vi "ExSetupROI.vi"() -> ()   [LabVIEW 2010]
uses:
  Open-Close Hardware/CamHandle.vi
panel:
  out "frames":u32=5341
  out "ADC Speed":u32=20000
  out "error out":errorcluster
  in  "error in (no error)":errorcluster
  in  "Timing Mode":u32(ring)=1 items=["N/A", "Timed Mode/Free run", "Trigger First (only PM)", "Strobed/Ext Sync", "Bulb Mode (PM only)", "Variable Timed mode (PM only)", "Flash Mode (only some PM)"]
  in  "x1":u32=1
  in  "x2":u32=256
  in  "y1":u32=1
  in  "y2":u32=256
  in  "x bin":u32=1
  in  "y bin":u32=1
  in  "min block":u32=2
  in  "Num Min Block":u32=5
  # "ExSetupROI.vi : This vi setups up 1 ROI (Region Of Interest)."
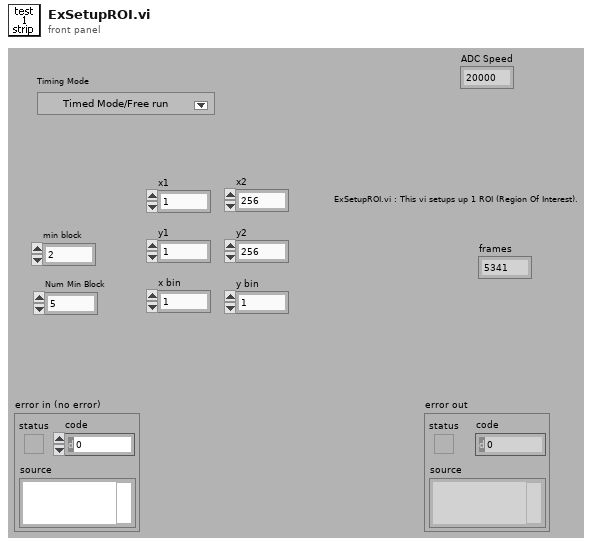
[diagram p1: front panel]
types:
  T1 = cluster{"x1":u32, "x2":u32, "x bin":u32, "y1":u32, "y2":u32, "y bin":u32}
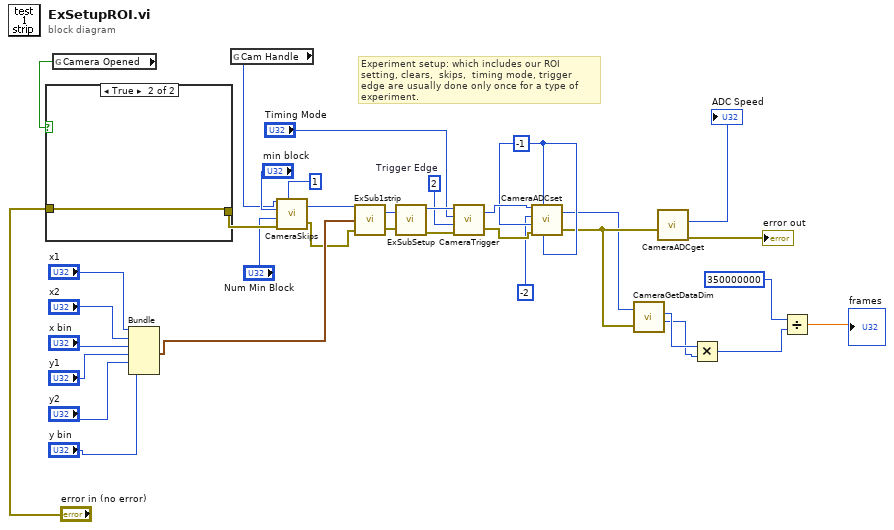
[diagram p0: block diagram]
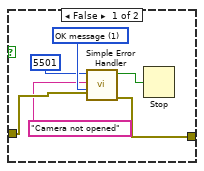
[diagram p2: hidden frame]
diagram:
  w29 = -1
  w33 = u32 2  # Trigger Edge
  # "Experiment setup: which includes our ROI setting, clears,  skips,  timing mode, trigger edge are usually done only once for a type of experiment."
  n1 = global read "CamHandle.vi" "Camera Opened"() -> (w32:bool)
  n2 = case shown="True" w32 {
    tunnel: "error in (no error)" -> [w40 w42]
    tunnel: [w39 w42] -> w19
    frame False {
      w41 = u16 1 items=["no dialog", "OK message", "continue or stop message"] ("type of dialog (OK msg:1)")
      n3 = call <vilib>:"Simple Error Handler.vi"("error code (no error:0)"=5501, "error source (\" \")"="Camera not opened", "type of dialog (OK msg:1)"=w41, "error in (no error)"=w40) -> ("error?"=w37:bool, "error out"=w39:errorcluster)  [unwired: 1 in, 3 out]
      n4 = Stop(stop? (T)=w37) -> ()
    }
    frame True {
    }
  }
  n5 = Bundle("x1"="x1", "x2"="x2", "x bin"="x bin", "y1"="y1", "y2"="y2", "y bin"="y bin") -> (w20:T1)  [unwired: 1 in]
  n6 = global read "CamHandle.vi" "Cam Handle"() -> (w12:u32)
  n7 = call <userlib>:"CameraSkips.vi"("Camera Handle"=w12, "Minimum Block Size"="min block", "Number of Minimum blocks"="Num Min Block", "error in"=w19, "Type of Skips"=1) -> ("Camera Handle"=w17:u32, "error out"=w18:errorcluster)
  n8 = call "ExSub1strip.vi"("error in (no error)"=w18, "strip 1"=w20, "Camera Handle"=w17) -> ("error out"=w27:errorcluster, "Camera Handle"=w13:u32)
  n9 = call "ExSubSetup.vi"("error in (no error)"=w27, "Camera Handle"=w13) -> ("error out"=w34:errorcluster, "Camera Handle"=w35:u32)
  n10 = call <userlib>:"CameraTrigger.vi"("error in"=w34, "Trigger Edge"=w33, "Timing Mode"="Timing Mode", "Camera Handle"=w35) -> ("error out"=w31:errorcluster, "Camera Handle"=w30:u32)
  n11 = call <userlib>:"CameraADCset.vi"("ADC offset"=w29, "Read Out port"=w29, "error in (no error)"=w31, "ADC Gain"=w29, "ADC Speed"=-2, "Camera Handle"=w30) -> ("error out"=w7:errorcluster, "Camera Handle"=w6:u32)
  n12 = call <userlib>:"CameraGetDataDim.vi"("Camera Handle"=w6, "error in"=w7) -> ("Xdim"=w5:u32, "Ydim"=w4:u32)  [unwired: 2 out]
  n13 = call <userlib>:"CameraADCget.vi"("error in (no error)"=w7) -> ("ADC Speed"=→"ADC Speed":i32, "error out"=→"error out":errorcluster)  [unwired: 1 in, 6 out]
  n14 = Multiply(x=w5, y=w4) -> (x*y=w2:u32)
  n15 = Divide(x=350000000, y=w2) -> (x/y=→"frames":dbl)
